vi "getCost.vi"(8 "error in (no error)":errorcluster, 11 "Meal in":refnum<class "Meal.lvclass">) -> (0 "error out":errorcluster, 2 "cost":dbl, 3 "Meal out":refnum<class "Meal.lvclass">)   [LabVIEW 2018, in "Meal.lvclass"]
uses:
  Meal.lvclass
  Meal.lvclass/Meal.ctl
  Item Class/Item.lvclass
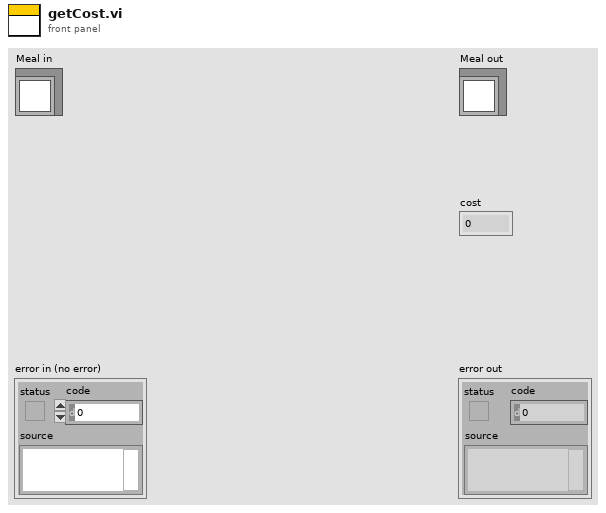
[diagram p1: front panel]
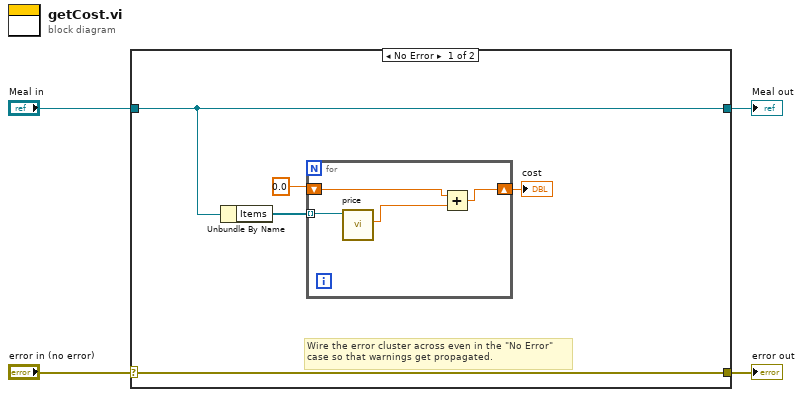
[diagram p0: block diagram]
diagram:
  n1 = case shown="No Error" "error in (no error)" {
    selector: "error in (no error)" -> [w9 w15]
    tunnel: [w9 w15] -> w3
    tunnel: [w8 w14] -> w1
    tunnel: "Meal in" -> [w8 w14]
    frame No Error {
      # "Wire the error cluster across even in the \"No Error\"\ncase so that warnings get propagated."
      n2 = Unbundle By Name(w8) -> ("Items"=w7:refnum<class "Item.lvclass">[])
      n3 = for {
        tunnel: w7 -> [w13] mode=indexing
        shift-right: [w10] -> w5
        shift-left: 0.0 -> [w11]
        n4 = call-dynamic "price.vi"("Item in"=w13) -> ("price"=w12:dbl)  [unwired: 8 in, 2 out]
        n5 = Add(x=w11, y=w12) -> (x+y=w10:dbl)
      }
      "cost" <- w5
    }
    frame Error {
    }
  }
  "error out" <- w3
  "Meal out" <- w1
